vi "WritingDataToDb.vi"() -> ()   [LabVIEW 2019]
uses:
  <vilib>/addons/database/Connection.llb/DB Tools Open Connec (String).vi
  <vilib>/addons/database/Auxilliary.llb/DB Tools Format Datetime String (Time Stamp).vi
  <vilib>/addons/database/NI_Database_API.lvlib
panel:
  in  "Connection Information":string
  in  "Number of Tests":dbl
  in  "Table Name":string
  out "Tesst Result Array":bool[](array[boolean])
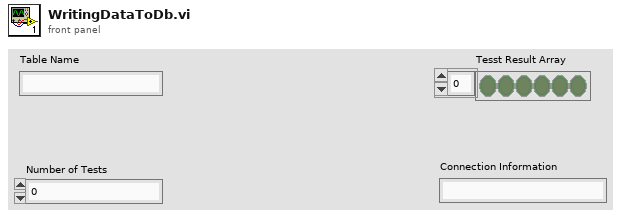
[diagram p1: front panel]
types:
  T1 = typedef "NI_Database_API.lvlib/Conn ObjectReference.ctl" = refnum<k1>
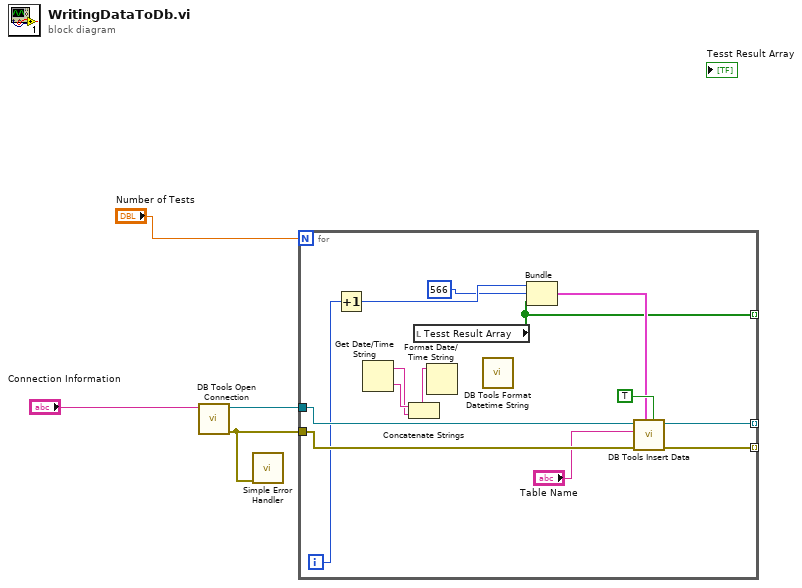
[diagram p0: block diagram]
diagram:
  n1 = call-poly <vilib>:"DB Tools Open Connection.vi"("connection information"="Connection Information") -> ("error out"=w1:errorcluster, "connection reference"=w2:T1)  [unwired: 7 in]
  n2 = call <vilib>:"Simple Error Handler.vi"("error in (no error)"=w1) -> ()  [unwired: 4 in, 5 out]
  n3 = for {
    N: "Number of Tests" -> [_]
    tunnel: w2 -> [w18]
    tunnel: w1 -> [w17]
    tunnel: [w10] -> _ mode=indexing
    tunnel: [w9] -> _ mode=indexing
    tunnel: [w8] -> _ mode=indexing
    i -> [w14]
    n4 = Increment(x=w14) -> (x+1=w13:i32)
    n5 = Get Date/Time String() -> (date string=w6:string, time string=w7:string)  [unwired: 3 in]
    n6 = Concatenate Strings(w7, w6) -> (w5:string)
    n7 = local read "Tesst Result Array"() -> (w8:bool[])
    n8 = Format Date/Time String(time format string (%c)=w5) -> ()  [unwired: 2 in, 1 out]
    n9 = call-poly <vilib>:"DB Tools Format Datetime String.vi"() -> ()  [unwired: 1 in, 1 out]
    n10 = Bundle(w13, 566, "Tesst Result Array"=w8) -> (w11:cluster{i32, i32, "Tesst Result Array":bool[]})  [unwired: 1 in]
    n11 = call <vilib>:"DB Tools Insert Data.vi"("create table? (F)"=TRUE, "data"=w11, "error in (no error)"=w17, "table"="Table Name", "connection reference"=w18) -> ("error out"=w9:errorcluster, "connection reference out"=w10:T1)  [unwired: 5 in]
  }
